vi "FPGA-Programm-05-17.vi"() -> ()   [LabVIEW 2017]
uses:
  <vilib>/LabVIEW Targets/FPGA/cRIO/shared/nicrio_ModuleControls/nicrio_cRIO-9871_BaudRateEnum.ctl
  <vilib>/LabVIEW Targets/FPGA/cRIO/shared/nicrio_ModuleControls/nicrio_cRIO-9871_DataBitsEnum.ctl
  <vilib>/LabVIEW Targets/FPGA/cRIO/shared/nicrio_ModuleControls/nicrio_cRIO-9871_ParityEnum.ctl
  <vilib>/LabVIEW Targets/FPGA/cRIO/shared/nicrio_ModuleControls/nicrio_cRIO-9871_StopBitsEnum.ctl
  <vilib>/LabVIEW Targets/FPGA/cRIO/shared/nicrio_ModuleControls/nicrio_cRIO-9871_FlowControlEnum.ctl
  <vilib>/rvi/Emulation/niFpgaSctlEmulationGetInTimedLoop.vi
  gvboolesch.vi
  <vilib>/rvi/Emulation/niFpgaProcessEmulError.vi
  <vilib>/rvi/Emulation/niFpgaGetClockAttributes.vi
  <vilib>/rvi/Emulation/niFpgaEmulationReportErrorSimple.vi
  <vilib>/rvi/Emulation/niFpgaCriticalErrorInLSC.vi
  <vilib>/rvi/eio/common/nirviEmuTemplateMethod_errors.vi
  <vilib>/eio/EIONode/EIONode.xnode
panel:
  in  "d1MainMach2":fxp<+/-,21,21> format="%.16g"
  in  "d0MainMach2":fxp<+/-,18,18> format="%.16g"
  in  "d1MainMach1":fxp<+/-,21,21> format="%.16g"
  in  "d0MainMach1":fxp<+/-,18,18> format="%.16g"
  in  "d1PreMach2":fxp<+/-,21,21> format="%.16g"
  in  "d0PreMach2":fxp<+/-,18,18> format="%.16g"
  in  "d1PreMach1":fxp<+/-,21,21> format="%.16g"
  in  "d0PreMach1":fxp<+/-,18,18> format="%.16g"
  in  "d1Trap2":fxp<+/-,21,21> format="%.16g"
  in  "d0Trap2":fxp<+/-,18,18> format="%.16g"
  in  "d1Trap1":fxp<+/-,21,21> format="%.16g"
  in  "d0Trap1":fxp<+/-,18,18> format="%.16g"
  in  "LHPulse(us)":T1
  in  "LHHeizen2?":T2
  in  "LHHeizen1?":T2
  in  "Mod6/DIOs":T3
  in  "Mod5/DIOs":T4
  in  "vor der Messung [us]Mach":u16=3000
  in  "Warten(us)":u16=5000
  out "MesswertTrap2":fxp<+/-,26,5> format="%.23g"
  in  "SetpointTrap2":fxp<+/-,26,5>
  in  "Heizen?Trap2":bool
  out "MesswertTrap1":fxp<+/-,26,5> format="%.23g"
  in  "SetpointTrap1":fxp<+/-,26,5>
  in  "USetp[V]MainMach2":fxp<+/-,26,5>
  in  "USetp[V]MainMach1":fxp<+/-,26,5>
  in  "Heizen?MainMach2":bool
  in  "Heizen?MainMach1":bool
  out "U[V]MainMach2":fxp<+/-,26,5> format="%.23g"
  out "U[V]MainMach1":fxp<+/-,26,5> format="%.23g"
  in  "USetp[V]PreMach2":fxp<+/-,26,5>
  in  "USetp[V]PreMach1":fxp<+/-,26,5>
  in  "Heizen?PreMach2":bool
  in  "Heizen?PreMach1":bool
  in  "Heizen?Trap1":bool
  in  "FIFO leer":bool
  in  "KonfigSeriell":T10
  out "U[V]PreMach1":fxp<+/-,26,5> format="%.23g"
  out "U[V]PreMach2":fxp<+/-,26,5> format="%.23g"
  in  "global stop":bool
  out "KonfigSeriellError":errorcluster
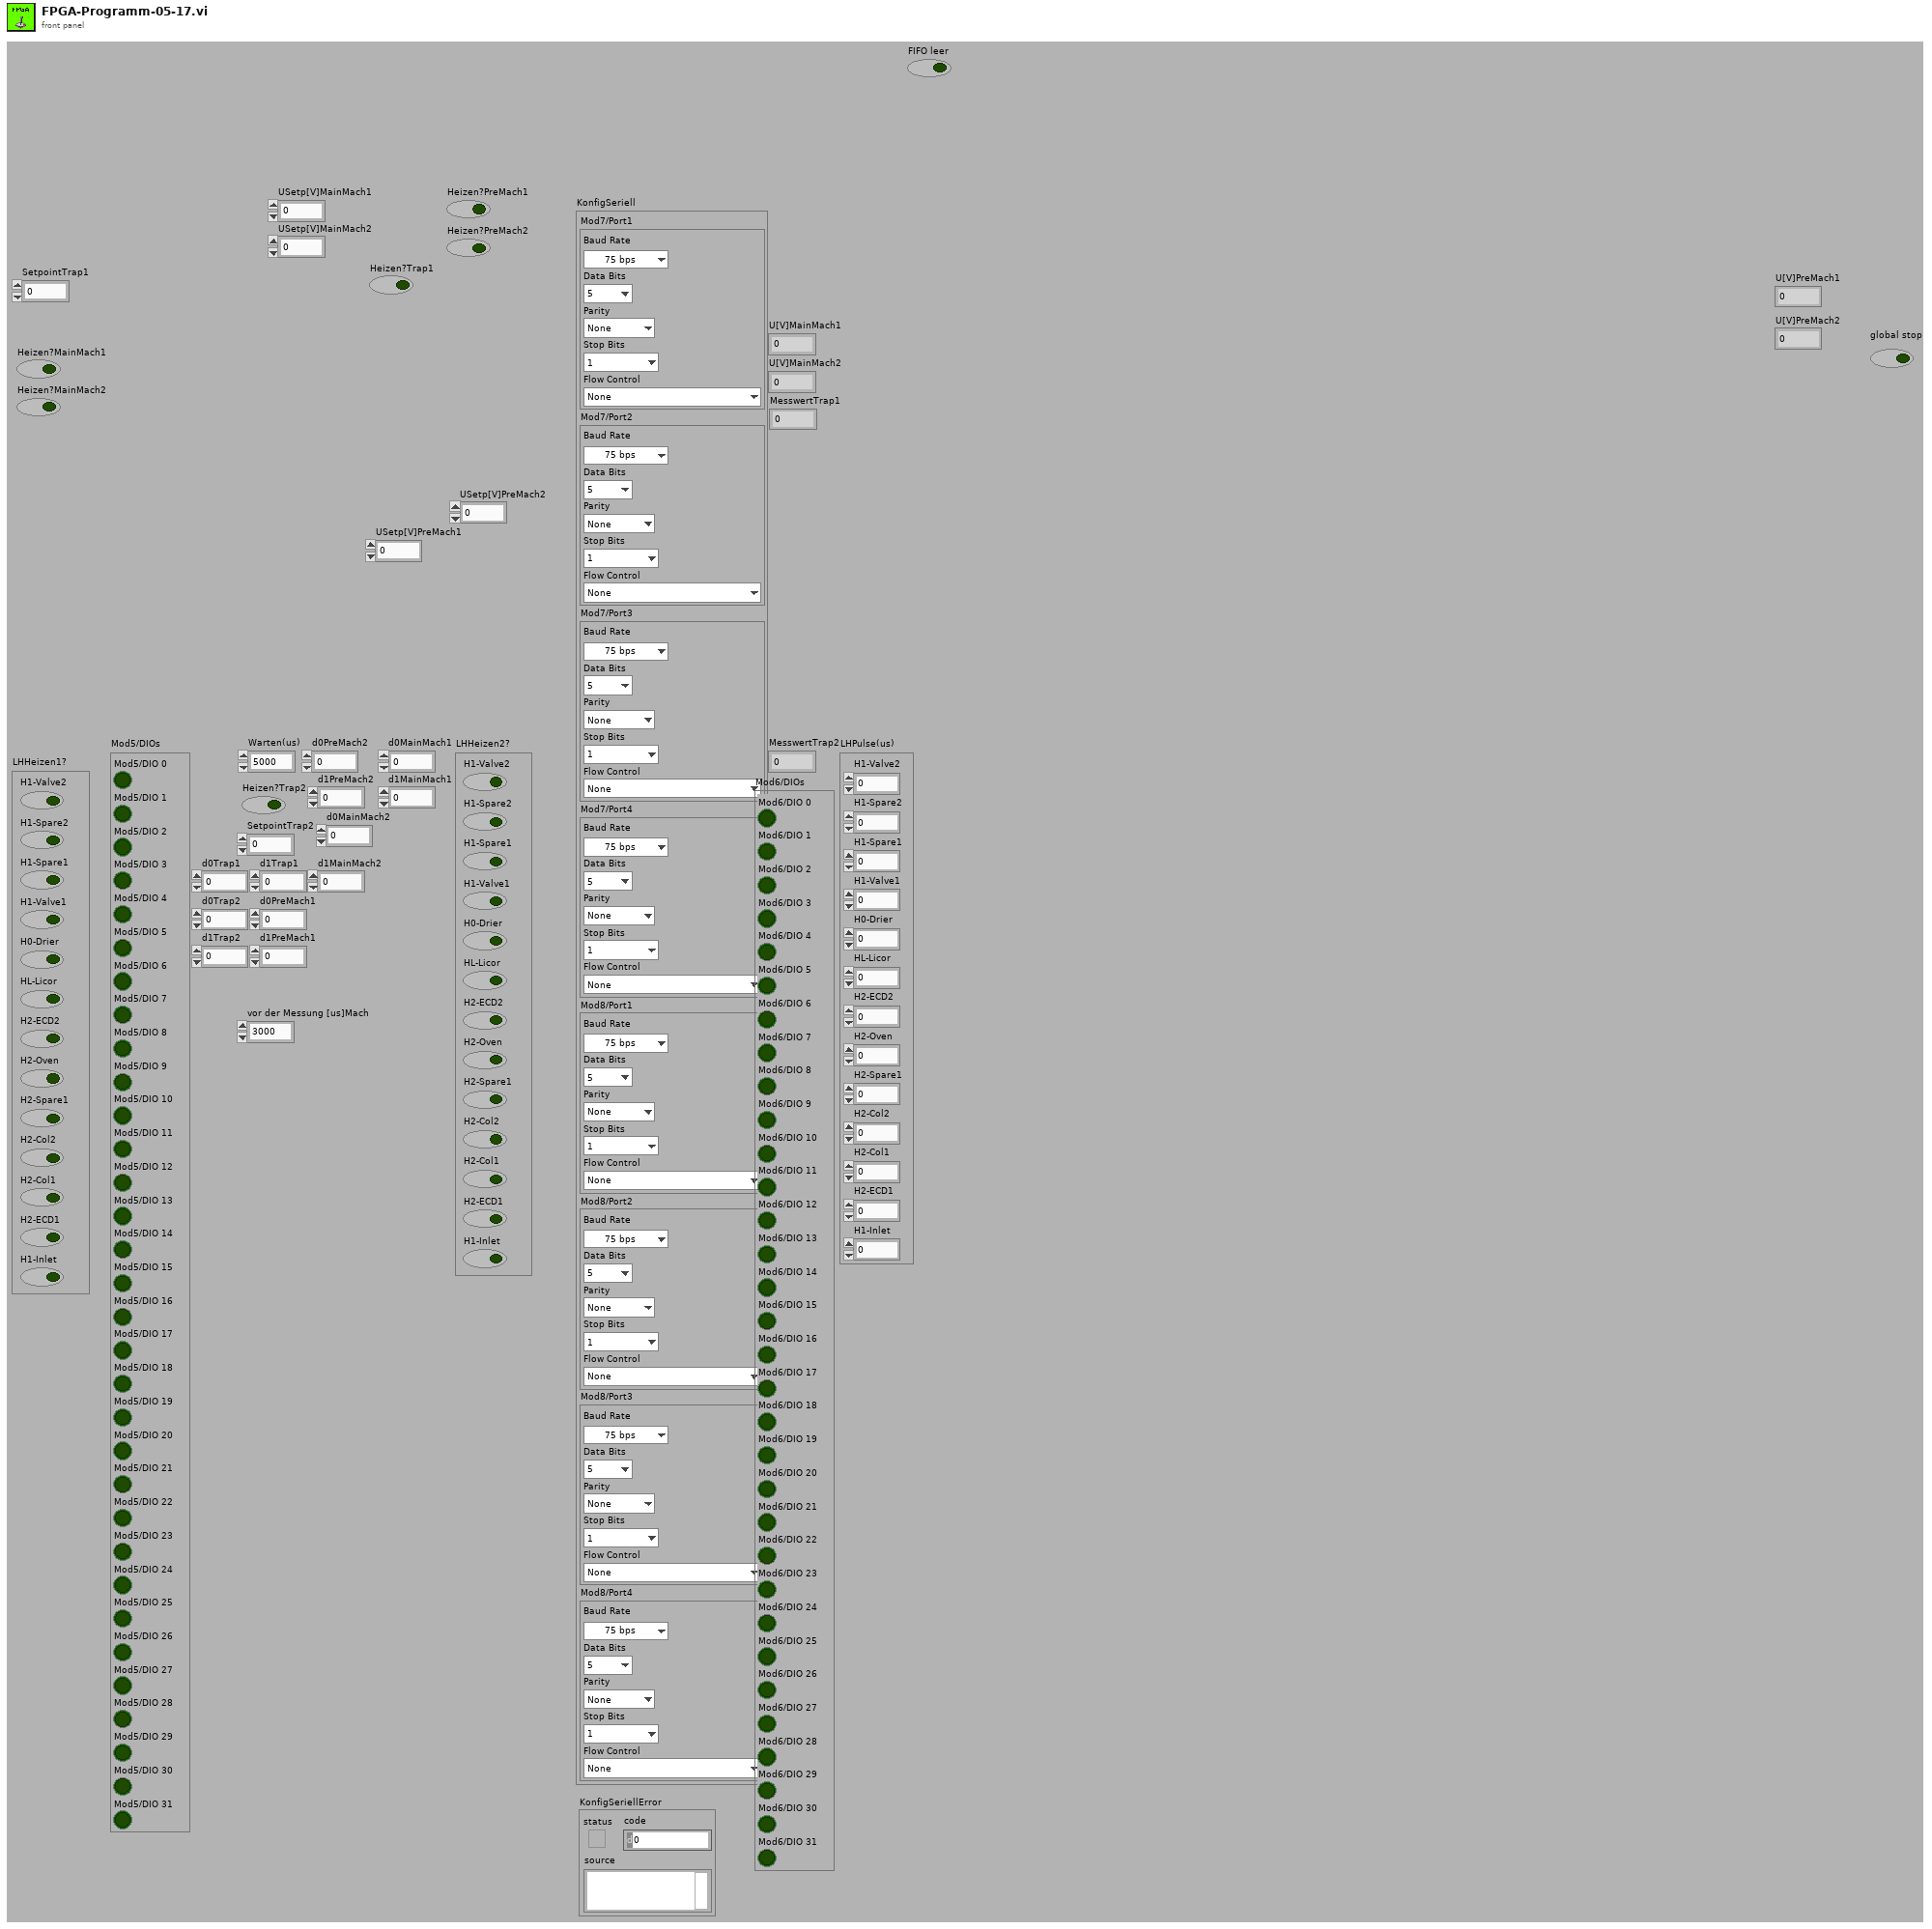
[diagram p1: front panel]
types:
  T1 = cluster{"H1-Valve2":u32, "H1-Spare2":u32, "H1-Spare1":u32, "H1-Valve1":u32, "H0-Drier":u32, "HL-Licor":u32, "H2-ECD2":u32, "H2-Oven":u32, "H2-Spare1":u32, "H2-Col2":u32, "H2-Col1":u32, "H2-ECD1":u32, "H1-Inlet":u32}
  T2 = cluster{"H1-Valve2":bool, "H1-Spare2":bool, "H1-Spare1":bool, "H1-Valve1":bool, "H0-Drier":bool, "HL-Licor":bool, "H2-ECD2":bool, "H2-Oven":bool, "H2-Spare1":bool, "H2-Col2":bool, "H2-Col1":bool, "H2-ECD1":bool, "H1-Inlet":bool}
  T3 = cluster{"Mod6/DIO 0":bool, "Mod6/DIO 1":bool, "Mod6/DIO 2":bool, "Mod6/DIO 3":bool, "Mod6/DIO 4":bool, "Mod6/DIO 5":bool, "Mod6/DIO 6":bool, "Mod6/DIO 7":bool, "Mod6/DIO 8":bool, "Mod6/DIO 9":bool, "Mod6/DIO 10":bool, "Mod6/DIO 11":bool, "Mod6/DIO 12":bool, "Mod6/DIO 13":bool, "Mod6/DIO 14":bool, "Mod6/DIO 15":bool, "Mod6/DIO 16":bool, "Mod6/DIO 17":bool, "Mod6/DIO 18":bool, "Mod6/DIO 19":bool, "Mod6/DIO 20":bool, "Mod6/DIO 21":bool, "Mod6/DIO 22":bool, "Mod6/DIO 23":bool, "Mod6/DIO 24":bool, "Mod6/DIO 25":bool, "Mod6/DIO 26":bool, "Mod6/DIO 27":bool, "Mod6/DIO 28":bool, "Mod6/DIO 29":bool, "Mod6/DIO 30":bool, "Mod6/DIO 31":bool}
  T4 = cluster{"Mod5/DIO 0":bool, "Mod5/DIO 1":bool, "Mod5/DIO 2":bool, "Mod5/DIO 3":bool, "Mod5/DIO 4":bool, "Mod5/DIO 5":bool, "Mod5/DIO 6":bool, "Mod5/DIO 7":bool, "Mod5/DIO 8":bool, "Mod5/DIO 9":bool, "Mod5/DIO 10":bool, "Mod5/DIO 11":bool, "Mod5/DIO 12":bool, "Mod5/DIO 13":bool, "Mod5/DIO 14":bool, "Mod5/DIO 15":bool, "Mod5/DIO 16":bool, "Mod5/DIO 17":bool, "Mod5/DIO 18":bool, "Mod5/DIO 19":bool, "Mod5/DIO 20":bool, "Mod5/DIO 21":bool, "Mod5/DIO 22":bool, "Mod5/DIO 23":bool, "Mod5/DIO 24":bool, "Mod5/DIO 25":bool, "Mod5/DIO 26":bool, "Mod5/DIO 27":bool, "Mod5/DIO 28":bool, "Mod5/DIO 29":bool, "Mod5/DIO 30":bool, "Mod5/DIO 31":bool}
  T5 = typedef "nicrio_cRIO-9871_BaudRateEnum.ctl" = enum16{"75 bps", "110 bps", "134 bps", "150 bps", "300 bps", "600 bps", "1200 bps", "1800 bps", "2400 bps", "4800 bps", "7200 bps", "9600 bps", "14.4 kbps", "19.2 kbps", "28.8 kbps", "38.4 kbps", "57.6 kbps", "115.2 kbps", "230.4 kbps", "460.8 kbps", "921.6 kbps"}
  T6 = typedef "nicrio_cRIO-9871_DataBitsEnum.ctl" = enum8{"5", "6", "7", "8"}
  T7 = typedef "nicrio_cRIO-9871_ParityEnum.ctl" = enum8{"None", "Odd", "Even", "Mark", "Space"}
  T8 = typedef "nicrio_cRIO-9871_StopBitsEnum.ctl" = enum8{"1", "1.5", "2"}
  T9 = typedef "nicrio_cRIO-9871_FlowControlEnum.ctl" = enum8{"None", "Software (XON / XOFF)", "Hardware (RTS / CTS)"}
  T10 = cluster{"Mod7/Port1":cluster{"Baud Rate":T5, "Data Bits":T6, "Parity":T7, "Stop Bits":T8, "Flow Control":T9}, "Mod7/Port2":cluster{"Baud Rate":T5, "Data Bits":T6, "Parity":T7, "Stop Bits":T8, "Flow Control":T9}, "Mod7/Port3":cluster{"Baud Rate":T5, "Data Bits":T6, "Parity":T7, "Stop Bits":T8, "Flow Control":T9}, "Mod7/Port4":cluster{"Baud Rate":T5, "Data Bits":T6, "Parity":T7, "Stop Bits":T8, "Flow Control":T9}, "Mod8/Port1":cluster{"Baud Rate":T5, "Data Bits":T6, "Parity":T7, "Stop Bits":T8, "Flow Control":T9}, "Mod8/Port2":cluster{"Baud Rate":T5, "Data Bits":T6, "Parity":T7, "Stop Bits":T8, "Flow Control":T9}, "Mod8/Port3":cluster{"Baud Rate":T5, "Data Bits":T6, "Parity":T7, "Stop Bits":T8, "Flow Control":T9}, "Mod8/Port4":cluster{"Baud Rate":T5, "Data Bits":T6, "Parity":T7, "Stop Bits":T8, "Flow Control":T9}}
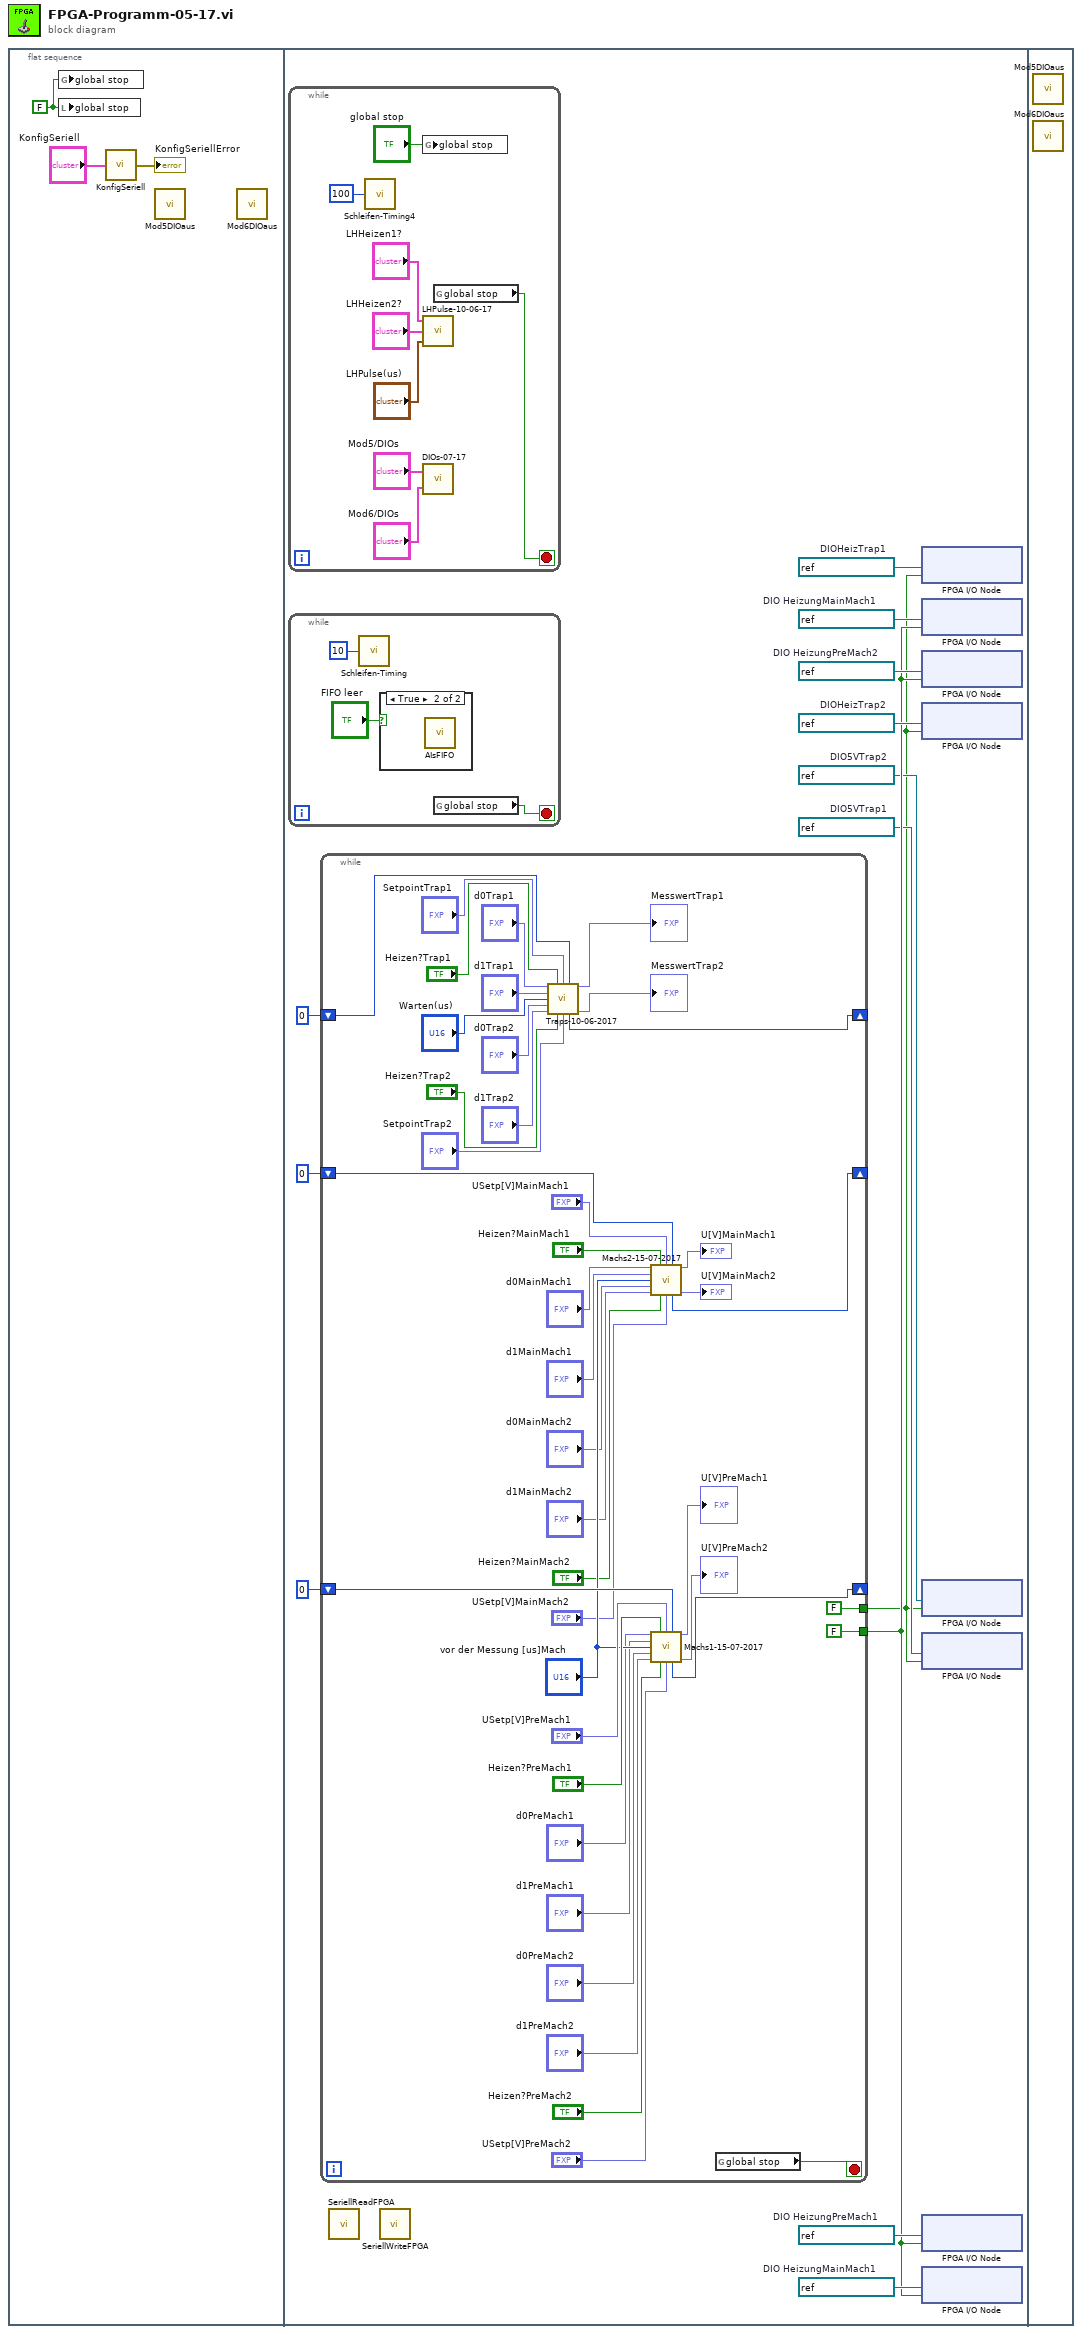
[diagram p0: block diagram]
diagram:
  n1 = flat-sequence {
    frame #0 {
      w1 = FALSE
      n2 = global write "gvboolesch.vi" "global stop"(w1) -> ()
      n3 = local write "global stop"(w1) -> ()
      n4 = call "KonfigSeriell.vi"("KonfigSeriell"="KonfigSeriell") -> ("KonfigSeriell"=→"KonfigSeriellError":errorcluster)
      n5 = call "Mod5DIOaus.vi"() -> ()  [unwired: 1 in]
      n6 = call "Mod6DIOaus.vi"() -> ()  [unwired: 1 in]
    }
    frame #1 {
      w8 = refnum<k21> "Mod6/DIO20"  # DIO5VTrap2
      w9 = refnum<k21> "Mod6/DIO21"  # DIO5VTrap1
      w11 = refnum<k21> "Mod6/DIO17"  # DIO HeizungMainMach1
      w12 = refnum<k21> "Mod6/DIO28"  # DIO HeizungMainMach1
      w13 = refnum<k21> "Mod6/DIO22"  # DIO HeizungPreMach2
      w14 = refnum<k21> "Mod6/DIO23"  # DIO HeizungPreMach1
      w15 = refnum<k21> "Mod6/DIO18"  # DIOHeizTrap2
      w16 = refnum<k21> "Mod6/DIO19"  # DIOHeizTrap1
      n7 = while {
        stop <- w25 stop-if-true
        n8 = call "Schleifen-Timing4"("Count(mSec)"=u8 100) -> ()  [unwired: 1 out]
        n9 = global write "gvboolesch.vi" "global stop"("global stop") -> ()
        n10 = call "LHPulse-10-06-17.vi"("LHPulse(us)"="LHPulse(us)", "LHHeizen2?"="LHHeizen2?", "LHHeizen1?"="LHHeizen1?") -> ()  [unwired: 1 in]
        n11 = call "DIOs-07-17.vi"("Mod6/DIOs"="Mod6/DIOs", "Mod5/DIOs"="Mod5/DIOs") -> ()  [unwired: 3 in]
        n12 = global read "gvboolesch.vi" "global stop"() -> (w25:bool)
      }
      n13 = while {
        stop <- w19 stop-if-true
        n14 = call "Schleifen-Timing"("Count(mSec)"=u8 10) -> ()  [unwired: 1 out]
        n15 = case shown="True" "FIFO leer" {
          frame False {
          }
          frame True {
            n16 = call "AIsFIFO.vi"() -> ()  [unwired: 12 in]
          }
        }
        n17 = global read "gvboolesch.vi" "global stop"() -> (w19:bool)
      }
      n18 = while {
        tunnel: [FALSE] -> w10
        shift-right: [w64] -> _
        shift-left: u32 0 ("Register->") -> [w63]
        shift-right: [w51] -> _
        shift-left: u32 0 ("Register->") -> [w50]
        tunnel: [FALSE ("I/O Item")] -> w5
        shift-right: [w28] -> _
        shift-left: u32 0 ("Register->") -> [w29]
        stop <- w68 stop-if-true
        n19 = call "Traps-10-06-2017.vi"("d0Trap1"="d0Trap1", "heizenTrap1"="Heizen?Trap1", "U_SPTrap1"="SetpointTrap1", "->Register"=w29, "d1Trap1"="d1Trap1", "Warten(uSec)"="Warten(us)", "d0Trap2"="d0Trap2", "d1Trap2"="d1Trap2", "heizenTrap2"="Heizen?Trap2", "U_SPTrap2"="SetpointTrap2") -> ("U_MWTrap1"=→"MesswertTrap1":fxp<+/-,26,5>, "Register->"=w28:u32, "U_MWTrap2"=→"MesswertTrap2":fxp<+/-,26,5>)  [unwired: 3 in]
        n20 = call "Machs2-15-07-2017.vi"("d0Mach1"="d0MainMach1", "heizenMach1"="Heizen?MainMach1", "U_SPMach1"="USetp[V]MainMach1", "->Register"=w50, "d1Mach1"="d1MainMach1", "Warten(uSec)"="vor der Messung [us]Mach", "d0Mach2"="d0MainMach2", "d1Mach2"="d1MainMach2", "heizenMach2"="Heizen?MainMach2", "U_SPMach2"="USetp[V]MainMach2") -> ("U_MWMach1"=→"U[V]MainMach1":fxp<+/-,26,5>, "Register->"=w51:u32, "U_MWMach2"=→"U[V]MainMach2":fxp<+/-,26,5>)  [unwired: 3 in]
        n21 = call "Machs1-15-07-2017.vi"("d0Mach1"="d0PreMach1", "heizenMach1"="Heizen?PreMach1", "U_SPMach1"="USetp[V]PreMach1", "->Register"=w63, "d1Mach1"="d1PreMach1", "Warten(uSec)"="vor der Messung [us]Mach", "d0Mach2"="d0PreMach2", "d1Mach2"="d1PreMach2", "heizenMach2"="Heizen?PreMach2", "U_SPMach2"="USetp[V]PreMach2") -> ("U_MWMach1"=→"U[V]PreMach1":fxp<+/-,26,5>, "Register->"=w64:u32, "U_MWMach2"=→"U[V]PreMach2":fxp<+/-,26,5>)  [unwired: 3 in]
        n22 = global read "gvboolesch.vi" "global stop"() -> (w68:bool)
      }
      n23 = call "SeriellReadFPGA.vi"() -> ()  [unwired: 12 in]
      n24 = call "SeriellWriteFPGA.vi"() -> ()  [unwired: 12 in]
      n25 = xnode "FPGA I/O Node"("I/O-Objekt"=w5, "FPGA-I/O (Eingang)"=w16) -> ()  [unwired: 1 out]
      n26 = xnode "FPGA I/O Node"("I/O-Objekt"=w10, "FPGA-I/O (Eingang)"=w12) -> ()  [unwired: 1 out]
      n27 = xnode "FPGA I/O Node"("I/O-Objekt"=w10, "FPGA-I/O (Eingang)"=w13) -> ()  [unwired: 1 out]
      n28 = xnode "FPGA I/O Node"("I/O-Objekt"=w5, "FPGA-I/O (Eingang)"=w15) -> ()  [unwired: 1 out]
      n29 = xnode "FPGA I/O Node"("I/O-Objekt"=w5, "FPGA-I/O (Eingang)"=w8) -> ()  [unwired: 1 out]
      n30 = xnode "FPGA I/O Node"("I/O-Objekt"=w5, "FPGA-I/O (Eingang)"=w9) -> ()  [unwired: 1 out]
      n31 = xnode "FPGA I/O Node"("I/O-Objekt"=w10, "FPGA-I/O (Eingang)"=w14) -> ()  [unwired: 1 out]
      n32 = xnode "FPGA I/O Node"("I/O-Objekt"=w10, "FPGA-I/O (Eingang)"=w11) -> ()  [unwired: 1 out]
    }
    frame #2 {
      n33 = call "Mod5DIOaus.vi"() -> ()  [unwired: 1 in]
      n34 = call "Mod6DIOaus.vi"() -> ()  [unwired: 1 in]
    }
  }
